vi "PicoScope6000aGetBlock.vi"(0 "handle in":i16, 1 "Acquisition Settings":T3 {"postTriggerSamples" format="%_6p"; "preTriggerSamples" format="%_6p"}, 2 "Buffer and Transfer Settings":T1 {"Down-Sample Mode" items=["None", "Aggregate", "Decimate", "Average"]; "Down Sample Ratio" step=1; "Samples" format="%_6p"}, 3 "enabled array":i16[](array[numeric]), 7 "stop IsReady":bool, 11 "error in (no error)":errorcluster) -> (4 "handle out":i16, 6 "Buffers (Max or non-aggregated)":T2, 10 "Min Buffers":T2, 12 "noOfSamples":u64, 14 "overflow":i16, 15 "error out":errorcluster)   [LabVIEW 2009]
doc: "GetBlock calls RunBlock and Sets up data buffers then calls GetValues"
uses:
  ps6000a.dll
panel:
  in  "PicoAction 2":u32(ring) items=["NONE", "CLEAR_ALL", "ADD", "CLEAR_THIS_DATA_BUFFER", "CLEAR_WAVEFORM_DATA_BUFFERS", "CLEAR_WAVEFORM_READ_DATA_BUFFERS"]
  in  "PicoAction 1":u32(ring) items=["NONE", "CLEAR_ALL", "ADD", "CLEAR_THIS_DATA_BUFFER", "CLEAR_WAVEFORM_DATA_BUFFERS", "CLEAR_WAVEFORM_READ_DATA_BUFFERS"]
  # "Pico Buffer Actions"
  # "Samples can be equal to or less\nTotal Pre and Post Trigger Samples"
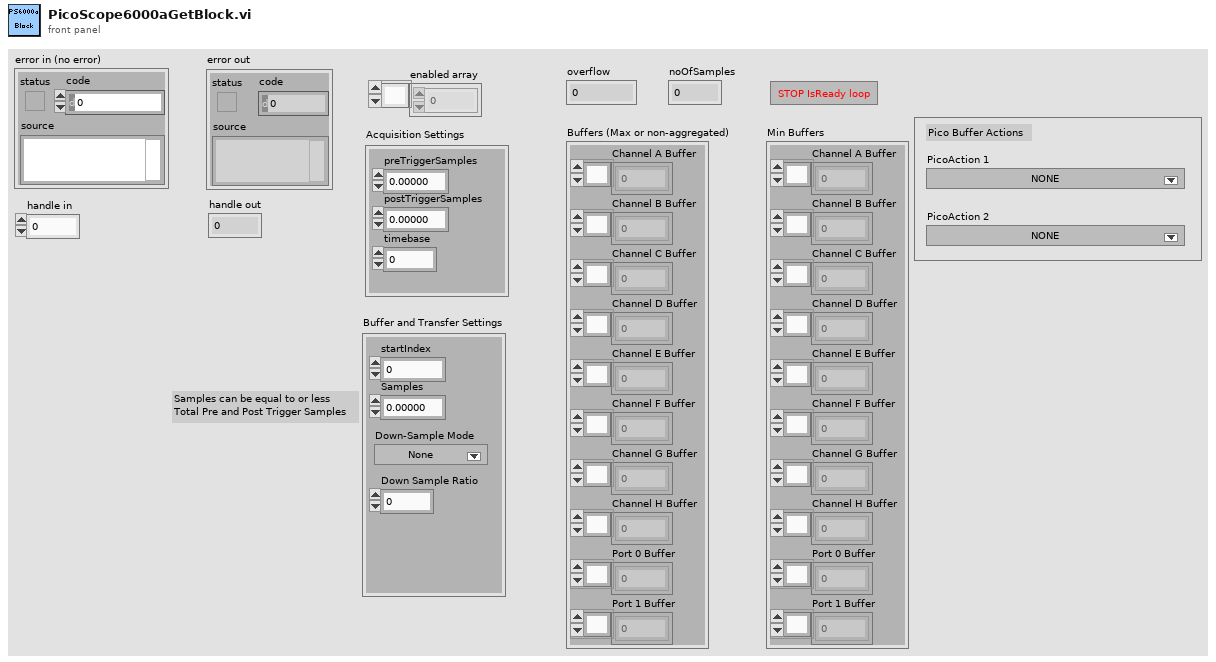
[diagram p1: front panel]
types:
  T1 = cluster{"startIndex":u64, "Samples":u64, "Down Sample Ratio":u64, "Down-Sample Mode":u32}
  T2 = cluster{"Channel A Buffer":i16[], "Channel B Buffer":i16[], "Channel C Buffer":i16[], "Channel D Buffer":i16[], "Channel E Buffer":i16[], "Channel F Buffer":i16[], "Channel G Buffer":i16[], "Channel H Buffer":i16[], "Port 0 Buffer":i16[], "Port 1 Buffer":i16[]}
  T3 = cluster{"preTriggerSamples":u64, "postTriggerSamples":u64, "timebase":u32}
  T4 = enum32{"PICO_INT8_T", "PICO_INT16_T", "PICO_INT32_T", "PICO_UINT32_T", "PICO_INT64_T", ""}
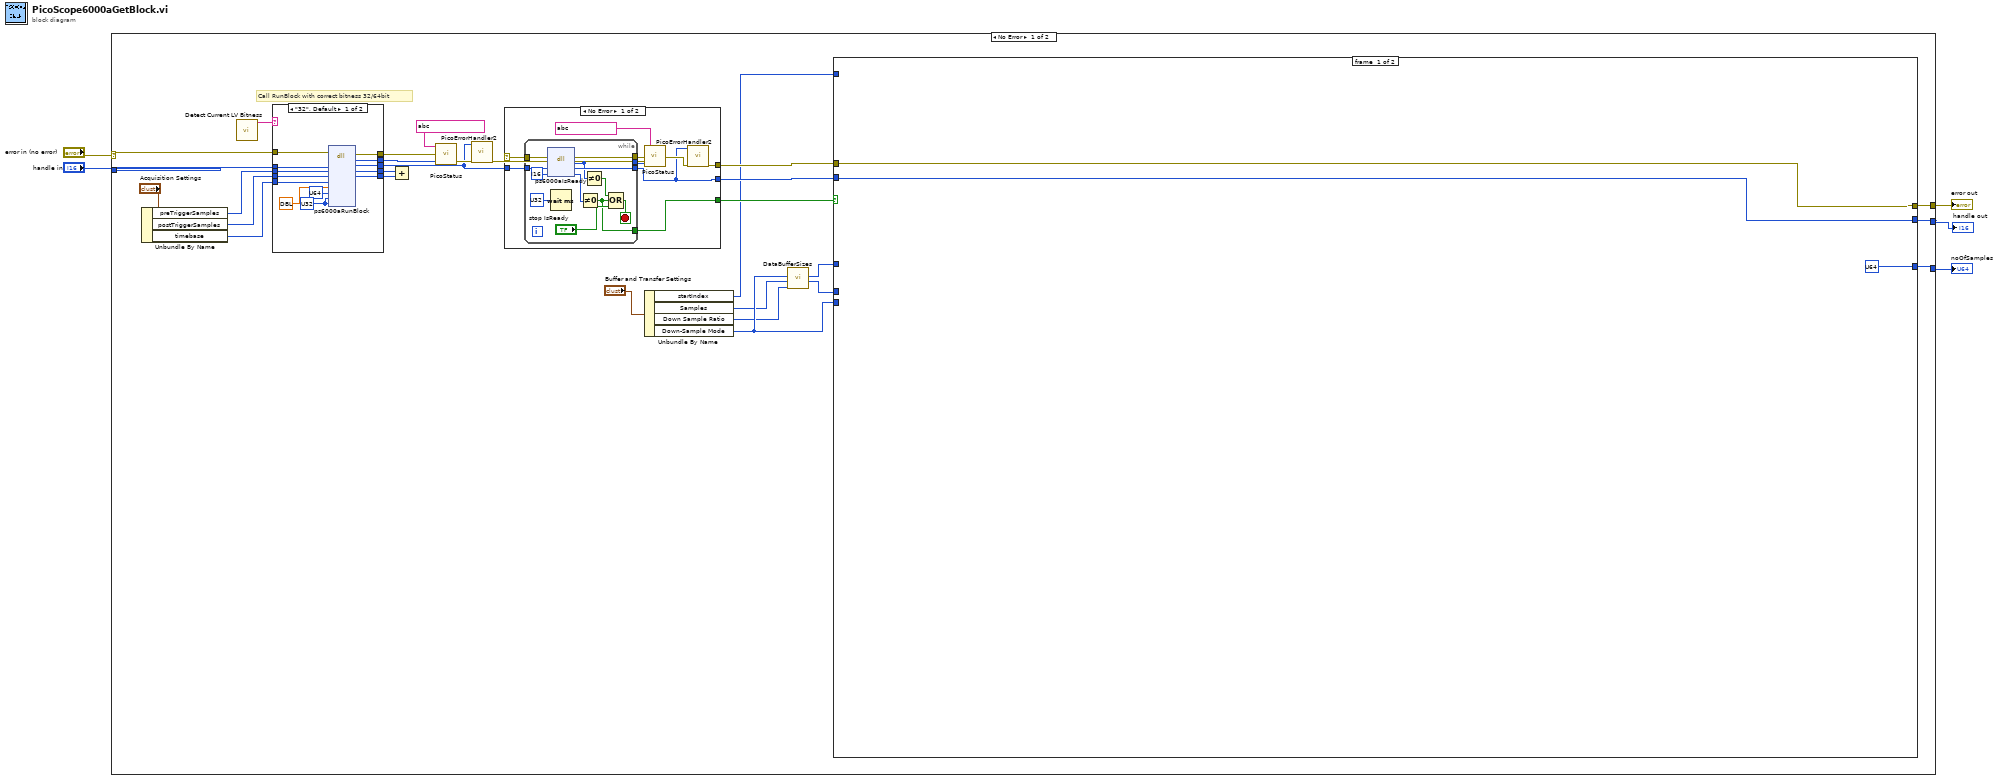
[diagram p0: block diagram]
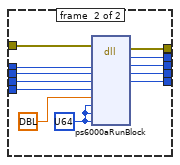
[diagram p2: hidden frame]
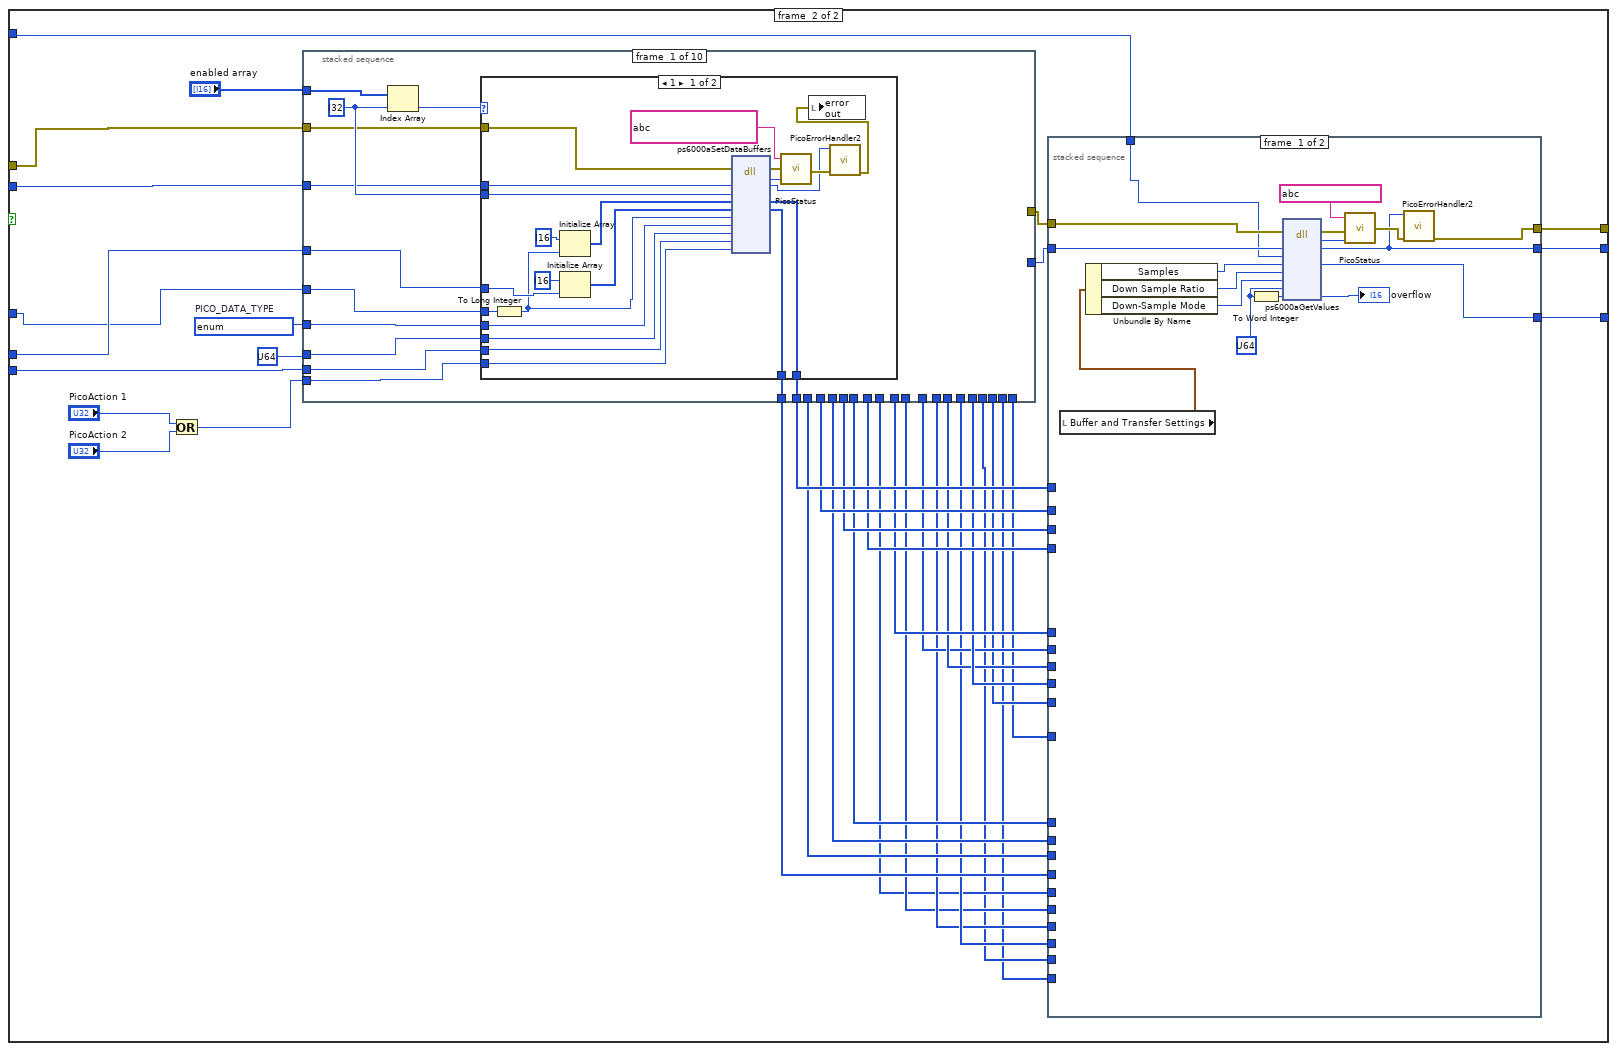
[diagram p3: hidden frame]
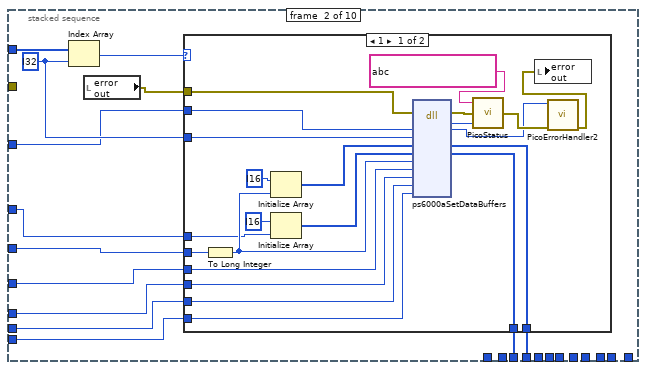
[diagram p5: hidden frame]
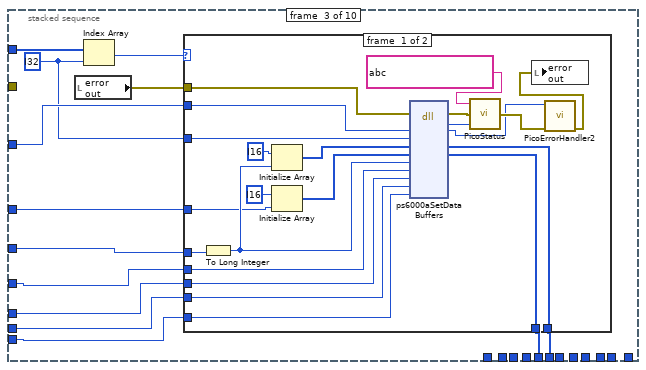
[diagram p7: hidden frame]
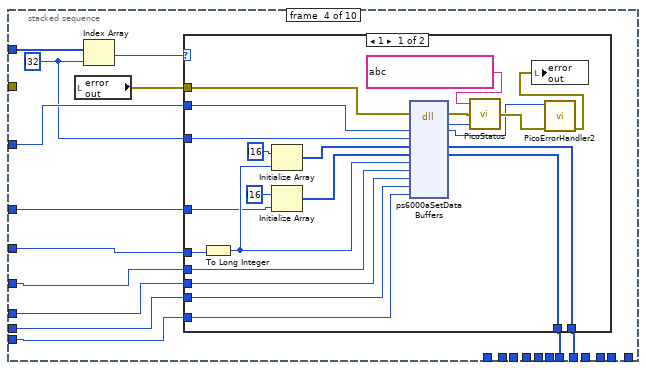
[diagram p9: hidden frame]
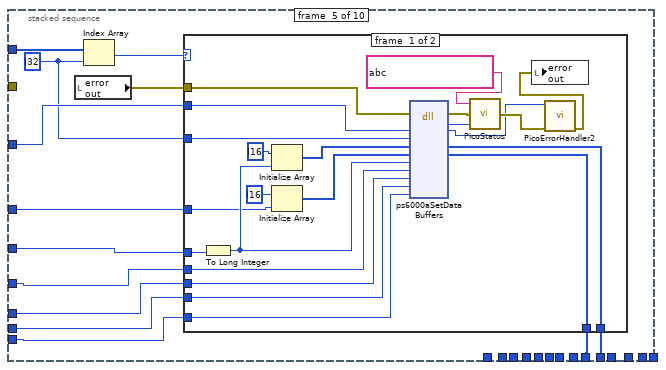
[diagram p11: hidden frame]
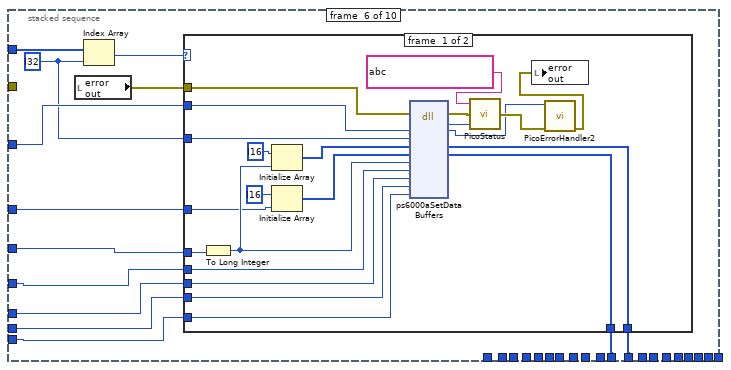
[diagram p13: hidden frame]
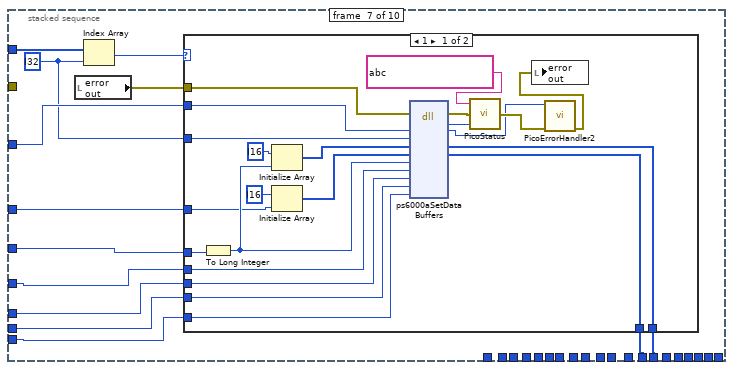
[diagram p15: hidden frame]
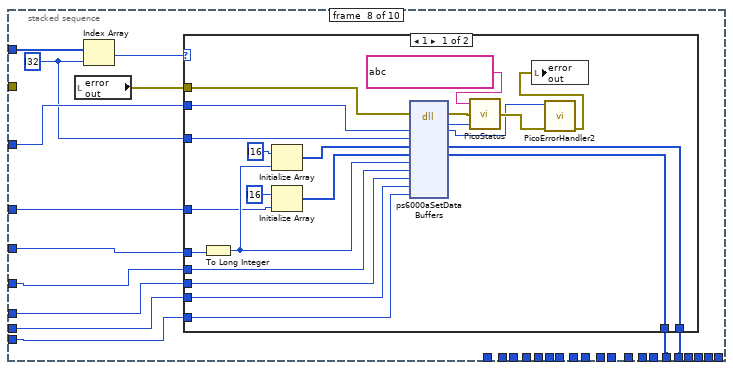
[diagram p17: hidden frame]
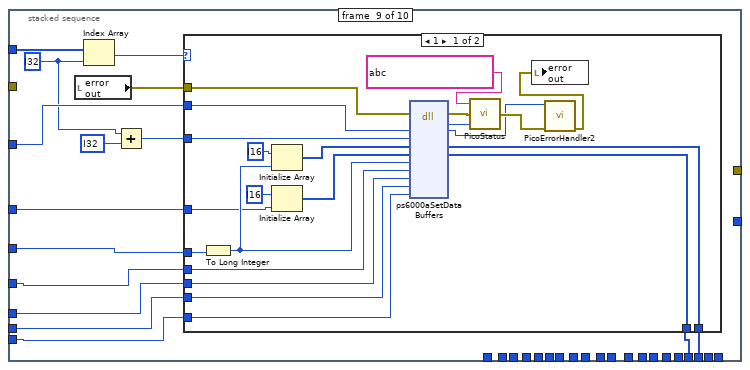
[diagram p19: hidden frame]
diagram:
  n1 = case shown="No Error" "error in (no error)" {
    selector: "error in (no error)" -> [w26 w524]
    tunnel: [w27 w524] -> w5
    tunnel: "handle in" -> [w25 w523]
    tunnel: [w24 w523] -> w4
    tunnel: [w19 u32 ? ("noOfSamples")] -> w1
    frame #0 {
      # "Call RunBlock with correct bitness 32/64bit"
      n2 = Unbundle By Name("Acquisition Settings") -> ("preTriggerSamples"=w23:u64, "postTriggerSamples"=w22:u64, "timebase"=w21:u32)
      n3 = call "Detect Current LV Bitness.vi"() -> ("bitness"=w11:string)  [unwired: 11 in]
      n4 = case shown="\"32\", Default" w11 {
        tunnel: [w46 w58] -> w33
        tunnel: [w45 w57] -> w32
        tunnel: [w44 w56] -> w30
        tunnel: [w43 w55] -> w29
        tunnel: w26 -> [w42 w54]
        tunnel: w25 -> [w41 w53]
        tunnel: w23 -> [w39 w51]
        tunnel: w22 -> [w38 w50]
        tunnel: w21 -> [w37 w49]
        tunnel: [w36 w48] -> w15
        frame #0 {
          w35 = u32 ? ("pParameter")
          n5 = dll-call lib="ps6000a.dll" fn="ps6000aRunBlock" ("ps3000.dll:_ps3000_open_unit@0")(error in=w42, "handle"=w41, "noOfPreTriggerSamples"=w39, "noOfPostTriggerSamples"=w38, "timebase"=w37, "timeIndisposedMs"=dbl ? ("pParameter"), "segmentIndex"=u64 ?, "lpReady"=w35, "pParameter"=w35) -> (error out=w43:errorcluster, "PICO_STATUS"=w44:u32, "handle"=w36:i16, "noOfPreTriggerSamples"=w46:u64, "noOfPostTriggerSamples"=w45:u64)  [unwired: 7 in, 1 out]
        }
        frame #1 {
          w47 = u64 ? ("pParameter")
          n6 = dll-call lib="ps6000a.dll" fn="ps6000aRunBlock" ("ps3000.dll:_ps3000_open_unit@0")(error in=w54, "handle"=w53, "noOfPreTriggerSamples"=w51, "noOfPostTriggerSamples"=w50, "timebase"=w49, "timeIndisposedMs"=dbl ? ("pParameter"), "segmentIndex"=w47, "lpReady"=w47, "pParameter"=w47) -> (error out=w55:errorcluster, "PICO_STATUS"=w56:u32, "handle"=w48:i16, "noOfPreTriggerSamples"=w58:u64, "noOfPostTriggerSamples"=w57:u64)  [unwired: 7 in, 1 out]
        }
      }
      n7 = Add(x=w33, y=w32) -> ()  [unwired: 1 out]
      n8 = call "PicoStatus.vi"("PICO STATUS"=w30, "error in"=w29, "source"=string ?) -> ("error out"=w20:errorcluster)
      n9 = call "PicoErrorHandler2.vi"("error in (no error)"=w20, "handle In"=w15) -> ("error out"=w18:errorcluster)  [unwired: 9 in]
      n10 = case shown="No Error" w18 {
        selector: w18 -> [w505 w520]
        tunnel: w15 -> [w506 w521]
        tunnel: [w499 w521] -> w16
        tunnel: [w500 w520] -> w17
        tunnel: [w498 bool ?] -> w14
        frame #0 {
          n11 = while {
            tunnel: [w518] -> w499
            tunnel: w506 -> [w517]
            tunnel: [w514] -> w503
            tunnel: w505 -> [w513]
            tunnel: [w512] -> w504
            tunnel: [w507] -> w498
            stop <- w516 stop-if-true
            n12 = dll-call lib="ps6000a.dll" fn="ps6000aIsReady" ("ps3000.dll:_ps3000_open_unit@0")(error in=w513, "handle"=w517, "ready"=i16 ?) -> (error out=w512:errorcluster, "PICO_STATUS"=w514:u32, "handle"=w518:i16, "ready"=w508:i16)  [unwired: 2 in, 1 out]
            n13 = Wait (ms)(milliseconds to wait=u32 ?) -> ()  [unwired: 1 out]
            n14 = Not Equal To 0?(x=w508) -> (x != 0?=w507:bool)
            n15 = Not Equal To 0?(x=w514) -> (x != 0?=w515:bool)
            n16 = Compound Arithmetic op=OR(w515, w507, "stop IsReady") -> (w516:bool)
          }
          n17 = call "PicoStatus.vi"("PICO STATUS"=w503, "error in"=w504, "source"=string ?) -> ("error out"=w501:errorcluster)
          n18 = call "PicoErrorHandler2.vi"("error in (no error)"=w501, "handle In"=w499) -> ("error out"=w500:errorcluster)  [unwired: 9 in]
        }
        frame #1 {
        }
      }
      n19 = Unbundle By Name("Buffer and Transfer Settings") -> ("startIndex"=w12:u64, "Samples"=w7:u64, "Down Sample Ratio"=w6:u64, "Down-Sample Mode"=w8:u32)
      n20 = call "DataBufferSizes.vi"("Down Sample Ratio"=w6, "Number of Samples"=w7, "Down-Sample Mode"=w8) -> ("min Buffer Size"=w9:i32, "Max Buffer Size"=w10:i32)  [unwired: 7 in]
      n21 = case shown="True" w14 {
        tunnel: [w59 w98] -> w27
        tunnel: [w60 w97] -> w24
        tunnel: [u64 ? ("noOfSamples") w96] -> w19
        tunnel: w17 -> [w59 w95]
        tunnel: w16 -> [w60 w94]
        tunnel: w9 -> [_ w67]
        tunnel: w10 -> [_ w62]
        tunnel: w8 -> [_ w93]
        tunnel: w12 -> [_ w68]
        frame #0 {
        }
        frame #1 {
          w69 = T4 ?  # PICO_DATA_TYPE
          n22 = Or(x="PicoAction 1", y="PicoAction 2") -> (x .or. y?=w70:u32)
          n23 = stacked-sequence {
            tunnel: "enabled array" -> [w110 w144 w180 w215 w250 w285 w320 w355 w392 w431]
            tunnel: w95 -> [w108 _ _ _ _ _ _ _ _ _]
            tunnel: w94 -> [w107 w143 w179 w214 w249 w284 w319 w354 w391 w430]
            tunnel: w62 -> [w106 w142 w170 w207 w242 w277 w312 w347 w385 w424]
            tunnel: w93 -> [w105 w136 w173 w210 w245 w280 w315 w350 w388 w427]
            tunnel: [w104 _ _ _ _ _ _ _ _ _] -> w91
            tunnel: [w103 _ _ _ _ _ _ _ _ _] -> w90
            tunnel: [_ w141 _ _ _ _ _ _ _ _] -> w89
            tunnel: [_ w140 _ _ _ _ _ _ _ _] -> w88
            tunnel: [_ _ w177 _ _ _ _ _ _ _] -> w87
            tunnel: [_ _ w176 _ _ _ _ _ _ _] -> w86
            tunnel: [_ _ _ w205 _ _ _ _ _ _] -> w85
            tunnel: [_ _ _ w204 _ _ _ _ _ _] -> w84
            tunnel: w69 -> [w102 w137 w171 w208 w243 w278 w313 w348 w386 w425]
            tunnel: u64 ? ("waveform") -> [w101 w135 w172 w209 w244 w279 w314 w349 w387 w426]
            tunnel: w70 -> [w100 w138 w174 w211 w246 w281 w316 w351 w389 w428]
            tunnel: [_ _ _ _ w239 _ _ _ _ _] -> w82
            tunnel: [_ _ _ _ _ _ _ w344 _ _] -> w81
            tunnel: [_ _ _ _ _ _ w309 _ _ _] -> w80
            tunnel: [_ _ _ _ _ w274 _ _ _ _] -> w79
            tunnel: [_ _ _ _ _ _ _ _ _ w422] -> w78
            tunnel: [_ _ _ _ _ _ _ _ _ w421] -> w77
            tunnel: [_ _ _ _ _ _ _ w345 _ _] -> w76
            tunnel: [_ _ _ _ _ _ w310 _ _ _] -> w75
            tunnel: [_ _ _ _ _ w275 _ _ _ _] -> w74
            tunnel: [_ _ _ _ w240 _ _ _ _ _] -> w73
            tunnel: w67 -> [w99 w134 w169 w206 w241 w276 w311 w346 w384 w423]
            tunnel: [_ _ _ _ _ _ _ _ w380 _] -> w66
            tunnel: [_ _ _ _ _ _ _ _ w379 _] -> w65
            tunnel: [_ _ _ _ _ _ _ _ _ w417] -> w64
            tunnel: [_ _ _ _ _ _ _ _ _ w416] -> w63
            frame #0 {
              w111 = i32 ? ("dimension size")
              n24 = Index Array(array=w110, index=w111) -> (element=w109:i16)
              n25 = case shown="1" w109 {
                tunnel: w111 -> [w128 _]
                tunnel: w108 -> [w133 _]
                tunnel: w107 -> [w130 _]
                tunnel: w106 -> [w113 _]
                tunnel: w105 -> [w122 _]
                tunnel: [w127 _] -> w104
                tunnel: [w126 _] -> w103
                tunnel: w102 -> [w121 _]
                tunnel: w101 -> [w120 _]
                tunnel: w100 -> [w119 _]
                tunnel: w99 -> [w115 _]
                frame #0 {
                  n26 = To Long Integer(number=w113) -> (32bit integer=w112:i32)
                  n27 = Initialize Array(i16 ? ("element"), w112) -> (w116:i16[])
                  n28 = Initialize Array(i16 ? ("element"), w115) -> (w114:i16[])
                  n29 = dll-call lib="ps6000a.dll" fn="ps6000aSetDataBuffers" ("ps3000.dll:_ps3000_open_unit@0")(error in=w133, "handle"=w130, "channel"=w128, "bufferMax"=w116, "bufferMin"=w114, "nSamples"=w112, "dataType"=w121, "waveform"=w120, "downSampleRatioMode"=w122, "action"=w119) -> (error out=w132:errorcluster, "PICO_STATUS"=w131:u32, "handle"=w123:i16, "bufferMax"=w126:i16[], "bufferMin"=w127:i16[])  [unwired: 8 in, 1 out]
                  n30 = call "PicoStatus.vi"("PICO STATUS"=w131, "error in"=w132, "source"=string ?) -> ("error out"=w125:errorcluster)
                  n31 = call "PicoErrorHandler2.vi"("error in (no error)"=w125, "handle In"=w123) -> ("error out"=w124:errorcluster)  [unwired: 9 in]
                  n32 = local write "error out"(w124) -> ()
                }
                frame #1 {
                }
              }
            }
            frame #1 {
              w146 = i32 ? ("dimension size")
              n33 = Index Array(array=w144, index=w146) -> (element=w145:i16)
              n34 = local read "error out"() -> (w139:errorcluster)
              n35 = case shown="1" w145 {
                tunnel: w146 -> [w148 _]
                tunnel: w139 -> [w162 _]
                tunnel: w143 -> [w147 _]
                tunnel: w135 -> [w157 _]
                tunnel: w142 -> [w152 _]
                tunnel: [w160 _] -> w141
                tunnel: [w161 _] -> w140
                tunnel: w138 -> [w159 _]
                tunnel: w137 -> [w156 _]
                tunnel: w136 -> [w158 _]
                tunnel: w134 -> [w151 _]
                frame #0 {
                  n36 = To Long Integer(number=w152) -> (32bit integer=w153:i32)
                  n37 = Initialize Array(i16 ? ("element"), w153) -> (w149:i16[])
                  n38 = Initialize Array(i16 ? ("element"), w151) -> (w150:i16[])
                  n39 = dll-call lib="ps6000a.dll" fn="ps6000aSetDataBuffers" ("ps3000.dll:_ps3000_open_unit@0")(error in=w162, "handle"=w147, "channel"=w148, "bufferMax"=w149, "bufferMin"=w150, "nSamples"=w153, "dataType"=w156, "waveform"=w157, "downSampleRatioMode"=w158, "action"=w159) -> (error out=w165:errorcluster, "PICO_STATUS"=w164:u32, "handle"=w163:i16, "bufferMax"=w161:i16[], "bufferMin"=w160:i16[])  [unwired: 8 in, 1 out]
                  n40 = call "PicoStatus.vi"("PICO STATUS"=w164, "error in"=w165, "source"=string ?) -> ("error out"=w167:errorcluster)
                  n41 = call "PicoErrorHandler2.vi"("error in (no error)"=w167, "handle In"=w163) -> ("error out"=w166:errorcluster)  [unwired: 9 in]
                  n42 = local write "error out"(w166) -> ()
                }
                frame #1 {
                }
              }
            }
            frame #2 {
              w175 = i32 ? ("dimension size")
              n43 = local read "error out"() -> (w178:errorcluster)
              n44 = Index Array(array=w180, index=w175) -> (element=w181:i16)
              n45 = case shown="0, Default" w181 {
                tunnel: w178 -> [w195 _]
                tunnel: w179 -> [w194 _]
                tunnel: [w196 _] -> w177
                tunnel: [w197 _] -> w176
                tunnel: w175 -> [w193 _]
                tunnel: w174 -> [w188 _]
                tunnel: w173 -> [w187 _]
                tunnel: w172 -> [w186 _]
                tunnel: w171 -> [w185 _]
                tunnel: w170 -> [w184 _]
                tunnel: w169 -> [w182 _]
                frame #0 {
                  n46 = To Long Integer(number=w184) -> (32bit integer=w183:i32)
                  n47 = Initialize Array(i16 ? ("element"), w183) -> (w190:i16[])
                  n48 = Initialize Array(i16 ? ("element"), w182) -> (w189:i16[])
                  n49 = dll-call lib="ps6000a.dll" fn="ps6000aSetDataBuffers" ("ps3000.dll:_ps3000_open_unit@0")(error in=w195, "handle"=w194, "channel"=w193, "bufferMax"=w190, "bufferMin"=w189, "nSamples"=w183, "dataType"=w185, "waveform"=w186, "downSampleRatioMode"=w187, "action"=w188) -> (error out=w200:errorcluster, "PICO_STATUS"=w199:u32, "handle"=w198:i16, "bufferMax"=w197:i16[], "bufferMin"=w196:i16[])  [unwired: 8 in, 1 out]
                  n50 = call "PicoStatus.vi"("PICO STATUS"=w199, "error in"=w200, "source"=string ?) -> ("error out"=w202:errorcluster)
                  n51 = call "PicoErrorHandler2.vi"("error in (no error)"=w202, "handle In"=w198) -> ("error out"=w201:errorcluster)  [unwired: 9 in]
                  n52 = local write "error out"(w201) -> ()
                }
                frame #1 {
                }
              }
            }
            frame #3 {
              w212 = i32 ? ("dimension size")
              n53 = local read "error out"() -> (w213:errorcluster)
              n54 = Index Array(array=w215, index=w212) -> (element=w216:i16)
              n55 = case shown="1" w216 {
                tunnel: w213 -> [w230 _]
                tunnel: w214 -> [w229 _]
                tunnel: [w231 _] -> w205
                tunnel: [w232 _] -> w204
                tunnel: w212 -> [w228 _]
                tunnel: w211 -> [w223 _]
                tunnel: w210 -> [w222 _]
                tunnel: w209 -> [w221 _]
                tunnel: w208 -> [w220 _]
                tunnel: w207 -> [w219 _]
                tunnel: w206 -> [w217 _]
                frame #0 {
                  n56 = To Long Integer(number=w219) -> (32bit integer=w218:i32)
                  n57 = Initialize Array(i16 ? ("element"), w218) -> (w225:i16[])
                  n58 = Initialize Array(i16 ? ("element"), w217) -> (w224:i16[])
                  n59 = dll-call lib="ps6000a.dll" fn="ps6000aSetDataBuffers" ("ps3000.dll:_ps3000_open_unit@0")(error in=w230, "handle"=w229, "channel"=w228, "bufferMax"=w225, "bufferMin"=w224, "nSamples"=w218, "dataType"=w220, "waveform"=w221, "downSampleRatioMode"=w222, "action"=w223) -> (error out=w235:errorcluster, "PICO_STATUS"=w234:u32, "handle"=w233:i16, "bufferMax"=w232:i16[], "bufferMin"=w231:i16[])  [unwired: 8 in, 1 out]
                  n60 = call "PicoStatus.vi"("PICO STATUS"=w234, "error in"=w235, "source"=string ?) -> ("error out"=w237:errorcluster)
                  n61 = call "PicoErrorHandler2.vi"("error in (no error)"=w237, "handle In"=w233) -> ("error out"=w236:errorcluster)  [unwired: 9 in]
                  n62 = local write "error out"(w236) -> ()
                }
                frame #1 {
                }
              }
            }
            frame #4 {
              w247 = i32 ? ("dimension size")
              n63 = local read "error out"() -> (w248:errorcluster)
              n64 = Index Array(array=w250, index=w247) -> (element=w251:i16)
              n65 = case shown="0, Default" w251 {
                tunnel: w248 -> [w265 _]
                tunnel: w249 -> [w264 _]
                tunnel: [w266 _] -> w240
                tunnel: [w267 _] -> w239
                tunnel: w247 -> [w263 _]
                tunnel: w246 -> [w258 _]
                tunnel: w245 -> [w257 _]
                tunnel: w244 -> [w256 _]
                tunnel: w243 -> [w255 _]
                tunnel: w242 -> [w254 _]
                tunnel: w241 -> [w252 _]
                frame #0 {
                  n66 = To Long Integer(number=w254) -> (32bit integer=w253:i32)
                  n67 = Initialize Array(i16 ? ("element"), w253) -> (w260:i16[])
                  n68 = Initialize Array(i16 ? ("element"), w252) -> (w259:i16[])
                  n69 = dll-call lib="ps6000a.dll" fn="ps6000aSetDataBuffers" ("ps3000.dll:_ps3000_open_unit@0")(error in=w265, "handle"=w264, "channel"=w263, "bufferMax"=w260, "bufferMin"=w259, "nSamples"=w253, "dataType"=w255, "waveform"=w256, "downSampleRatioMode"=w257, "action"=w258) -> (error out=w270:errorcluster, "PICO_STATUS"=w269:u32, "handle"=w268:i16, "bufferMax"=w267:i16[], "bufferMin"=w266:i16[])  [unwired: 8 in, 1 out]
                  n70 = call "PicoStatus.vi"("PICO STATUS"=w269, "error in"=w270, "source"=string ?) -> ("error out"=w272:errorcluster)
                  n71 = call "PicoErrorHandler2.vi"("error in (no error)"=w272, "handle In"=w268) -> ("error out"=w271:errorcluster)  [unwired: 9 in]
                  n72 = local write "error out"(w271) -> ()
                }
                frame #1 {
                }
              }
            }
            frame #5 {
              w282 = i32 ? ("dimension size")
              n73 = local read "error out"() -> (w283:errorcluster)
              n74 = Index Array(array=w285, index=w282) -> (element=w286:i16)
              n75 = case shown="0, Default" w286 {
                tunnel: w283 -> [w300 _]
                tunnel: w284 -> [w299 _]
                tunnel: [w301 _] -> w275
                tunnel: [w302 _] -> w274
                tunnel: w282 -> [w298 _]
                tunnel: w281 -> [w293 _]
                tunnel: w280 -> [w292 _]
                tunnel: w279 -> [w291 _]
                tunnel: w278 -> [w290 _]
                tunnel: w277 -> [w289 _]
                tunnel: w276 -> [w287 _]
                frame #0 {
                  n76 = To Long Integer(number=w289) -> (32bit integer=w288:i32)
                  n77 = Initialize Array(i16 ? ("element"), w288) -> (w295:i16[])
                  n78 = Initialize Array(i16 ? ("element"), w287) -> (w294:i16[])
                  n79 = dll-call lib="ps6000a.dll" fn="ps6000aSetDataBuffers" ("ps3000.dll:_ps3000_open_unit@0")(error in=w300, "handle"=w299, "channel"=w298, "bufferMax"=w295, "bufferMin"=w294, "nSamples"=w288, "dataType"=w290, "waveform"=w291, "downSampleRatioMode"=w292, "action"=w293) -> (error out=w305:errorcluster, "PICO_STATUS"=w304:u32, "handle"=w303:i16, "bufferMax"=w302:i16[], "bufferMin"=w301:i16[])  [unwired: 8 in, 1 out]
                  n80 = call "PicoStatus.vi"("PICO STATUS"=w304, "error in"=w305, "source"=string ?) -> ("error out"=w307:errorcluster)
                  n81 = call "PicoErrorHandler2.vi"("error in (no error)"=w307, "handle In"=w303) -> ("error out"=w306:errorcluster)  [unwired: 9 in]
                  n82 = local write "error out"(w306) -> ()
                }
                frame #1 {
                }
              }
            }
            frame #6 {
              w317 = i32 ? ("dimension size")
              n83 = local read "error out"() -> (w318:errorcluster)
              n84 = Index Array(array=w320, index=w317) -> (element=w321:i16)
              n85 = case shown="1" w321 {
                tunnel: w318 -> [w335 _]
                tunnel: w319 -> [w334 _]
                tunnel: [w336 _] -> w310
                tunnel: [w337 _] -> w309
                tunnel: w317 -> [w333 _]
                tunnel: w316 -> [w328 _]
                tunnel: w315 -> [w327 _]
                tunnel: w314 -> [w326 _]
                tunnel: w313 -> [w325 _]
                tunnel: w312 -> [w324 _]
                tunnel: w311 -> [w322 _]
                frame #0 {
                  n86 = To Long Integer(number=w324) -> (32bit integer=w323:i32)
                  n87 = Initialize Array(i16 ? ("element"), w323) -> (w330:i16[])
                  n88 = Initialize Array(i16 ? ("element"), w322) -> (w329:i16[])
                  n89 = dll-call lib="ps6000a.dll" fn="ps6000aSetDataBuffers" ("ps3000.dll:_ps3000_open_unit@0")(error in=w335, "handle"=w334, "channel"=w333, "bufferMax"=w330, "bufferMin"=w329, "nSamples"=w323, "dataType"=w325, "waveform"=w326, "downSampleRatioMode"=w327, "action"=w328) -> (error out=w340:errorcluster, "PICO_STATUS"=w339:u32, "handle"=w338:i16, "bufferMax"=w337:i16[], "bufferMin"=w336:i16[])  [unwired: 8 in, 1 out]
                  n90 = call "PicoStatus.vi"("PICO STATUS"=w339, "error in"=w340, "source"=string ?) -> ("error out"=w342:errorcluster)
                  n91 = call "PicoErrorHandler2.vi"("error in (no error)"=w342, "handle In"=w338) -> ("error out"=w341:errorcluster)  [unwired: 9 in]
                  n92 = local write "error out"(w341) -> ()
                }
                frame #1 {
                }
              }
            }
            frame #7 {
              w352 = i32 ? ("dimension size")
              n93 = local read "error out"() -> (w353:errorcluster)
              n94 = Index Array(array=w355, index=w352) -> (element=w356:i16)
              n95 = case shown="1" w356 {
                tunnel: w353 -> [w370 _]
                tunnel: w354 -> [w369 _]
                tunnel: [w371 _] -> w345
                tunnel: [w372 _] -> w344
                tunnel: w352 -> [w368 _]
                tunnel: w351 -> [w363 _]
                tunnel: w350 -> [w362 _]
                tunnel: w349 -> [w361 _]
                tunnel: w348 -> [w360 _]
                tunnel: w347 -> [w359 _]
                tunnel: w346 -> [w357 _]
                frame #0 {
                  n96 = To Long Integer(number=w359) -> (32bit integer=w358:i32)
                  n97 = Initialize Array(i16 ? ("element"), w358) -> (w365:i16[])
                  n98 = Initialize Array(i16 ? ("element"), w357) -> (w364:i16[])
                  n99 = dll-call lib="ps6000a.dll" fn="ps6000aSetDataBuffers" ("ps3000.dll:_ps3000_open_unit@0")(error in=w370, "handle"=w369, "channel"=w368, "bufferMax"=w365, "bufferMin"=w364, "nSamples"=w358, "dataType"=w360, "waveform"=w361, "downSampleRatioMode"=w362, "action"=w363) -> (error out=w375:errorcluster, "PICO_STATUS"=w374:u32, "handle"=w373:i16, "bufferMax"=w372:i16[], "bufferMin"=w371:i16[])  [unwired: 8 in, 1 out]
                  n100 = call "PicoStatus.vi"("PICO STATUS"=w374, "error in"=w375, "source"=string ?) -> ("error out"=w377:errorcluster)
                  n101 = call "PicoErrorHandler2.vi"("error in (no error)"=w377, "handle In"=w373) -> ("error out"=w376:errorcluster)  [unwired: 9 in]
                  n102 = local write "error out"(w376) -> ()
                }
                frame #1 {
                }
              }
            }
            frame #8 {
              w381 = i32 ? ("dimension size")
              n103 = local read "error out"() -> (w390:errorcluster)
              n104 = Index Array(array=w392, index=w381) -> (element=w393:i16)
              n105 = Add(x=w381, y=i32 ?) -> (x+y=w382:i32)
              n106 = case shown="1" w393 {
                tunnel: w390 -> [w407 _]
                tunnel: w391 -> [w406 _]
                tunnel: [w408 _] -> w380
                tunnel: [w409 _] -> w379
                tunnel: w382 -> [w405 _]
                tunnel: w389 -> [w400 _]
                tunnel: w388 -> [w399 _]
                tunnel: w387 -> [w398 _]
                tunnel: w386 -> [w397 _]
                tunnel: w385 -> [w396 _]
                tunnel: w384 -> [w394 _]
                frame #0 {
                  n107 = To Long Integer(number=w396) -> (32bit integer=w395:i32)
                  n108 = Initialize Array(i16 ? ("element"), w395) -> (w402:i16[])
                  n109 = Initialize Array(i16 ? ("element"), w394) -> (w401:i16[])
                  n110 = dll-call lib="ps6000a.dll" fn="ps6000aSetDataBuffers" ("ps3000.dll:_ps3000_open_unit@0")(error in=w407, "handle"=w406, "channel"=w405, "bufferMax"=w402, "bufferMin"=w401, "nSamples"=w395, "dataType"=w397, "waveform"=w398, "downSampleRatioMode"=w399, "action"=w400) -> (error out=w412:errorcluster, "PICO_STATUS"=w411:u32, "handle"=w410:i16, "bufferMax"=w409:i16[], "bufferMin"=w408:i16[])  [unwired: 8 in, 1 out]
                  n111 = call "PicoStatus.vi"("PICO STATUS"=w411, "error in"=w412, "source"=string ?) -> ("error out"=w414:errorcluster)
                  n112 = call "PicoErrorHandler2.vi"("error in (no error)"=w414, "handle In"=w410) -> ("error out"=w413:errorcluster)  [unwired: 9 in]
                  n113 = local write "error out"(w413) -> ()
                }
                frame #1 {
                }
              }
            }
            frame #9 {
              w419 = i32 ? ("dimension size")
              n114 = local read "error out"() -> (w429:errorcluster)
              n115 = Index Array(array=w431, index=w419) -> (element=w432:i16)
              n116 = Add(x=w419, y=i32 ?) -> (x+y=w420:i32)
              n117 = case shown="1" w432 {
                tunnel: w429 -> [w448 w456]
                tunnel: w430 -> [w447 w455]
                tunnel: [w449 _] -> w417
                tunnel: [w450 _] -> w416
                tunnel: w420 -> [w446 _]
                tunnel: w428 -> [w441 _]
                tunnel: w427 -> [w440 _]
                tunnel: w426 -> [w439 _]
                tunnel: w425 -> [w438 _]
                tunnel: w424 -> [w437 _]
                tunnel: w423 -> [w435 _]
                tunnel: [w434 w456] -> w422
                tunnel: [w433 w455] -> w421
                frame #0 {
                  n118 = To Long Integer(number=w437) -> (32bit integer=w436:i32)
                  n119 = Initialize Array(i16 ? ("element"), w436) -> (w443:i16[])
                  n120 = Initialize Array(i16 ? ("element"), w435) -> (w442:i16[])
                  n121 = dll-call lib="ps6000a.dll" fn="ps6000aSetDataBuffers" ("ps3000.dll:_ps3000_open_unit@0")(error in=w448, "handle"=w447, "channel"=w446, "bufferMax"=w443, "bufferMin"=w442, "nSamples"=w436, "dataType"=w438, "waveform"=w439, "downSampleRatioMode"=w440, "action"=w441) -> (error out=w452:errorcluster, "PICO_STATUS"=w451:u32, "handle"=w433:i16, "bufferMax"=w450:i16[], "bufferMin"=w449:i16[])  [unwired: 8 in, 1 out]
                  n122 = call "PicoStatus.vi"("PICO STATUS"=w451, "error in"=w452, "source"=string ?) -> ("error out"=w453:errorcluster)
                  n123 = call "PicoErrorHandler2.vi"("error in (no error)"=w453, "handle In"=w433) -> ("error out"=w434:errorcluster)  [unwired: 9 in]
                }
                frame #1 {
                }
              }
            }
          }
          n124 = stacked-sequence {
            tunnel: [w462 _] -> w98
            tunnel: [w460 _] -> w97
            tunnel: [w465 _] -> w96
            tunnel: w91 -> [_ w486]
            tunnel: w90 -> [_ w497]
            tunnel: w89 -> [_ w487]
            tunnel: w88 -> [_ w496]
            tunnel: w87 -> [_ w488]
            tunnel: w86 -> [_ w495]
            tunnel: w85 -> [_ w489]
            tunnel: w84 -> [_ w494]
            tunnel: w78 -> [w464 _]
            tunnel: w77 -> [w463 _]
            tunnel: w82 -> [_ w493]
            tunnel: w81 -> [_ w492]
            tunnel: w80 -> [_ w491]
            tunnel: w79 -> [_ w490]
            tunnel: w76 -> [_ w485]
            tunnel: w75 -> [_ w484]
            tunnel: w74 -> [_ w483]
            tunnel: w73 -> [_ w482]
            tunnel: w68 -> [w457 _]
            tunnel: w66 -> [_ w481]
            tunnel: w65 -> [_ w480]
            tunnel: w64 -> [_ w479]
            tunnel: w63 -> [_ w478]
            frame #0 {
              w472 = u64 ? ("overflow")
              n125 = local read "Buffer and Transfer Settings"() -> (w459:T1)
              n126 = Unbundle By Name(w459) -> ("Samples"=w458:u64, "Down Sample Ratio"=w468:u64, "Down-Sample Mode"=w467:u32)
              n127 = To Word Integer(number=w472) -> (16bit integer=w466:i16)
              n128 = dll-call lib="ps6000a.dll" fn="ps6000aGetValues" ("ps3000.dll:_ps3000_open_unit@0")(error in=w464, "handle"=w463, "startIndex"=w457, "noOfSamples"=w458, "downSampleRatio"=w468, "downSampleRatioMode"=w467, "segmentIndex"=w472, "overflow"=w466) -> (error out=w470:errorcluster, "PICO_STATUS"=w471:u32, "handle"=w460:i16, "noOfSamples"=w465:u64, "overflow"=→"overflow":i16)  [unwired: 6 in, 1 out]
              n129 = call "PicoStatus.vi"("PICO STATUS"=w471, "error in"=w470, "source"=string ?) -> ("error out"=w461:errorcluster)
              n130 = call "PicoErrorHandler2.vi"("error in (no error)"=w461, "handle In"=w460) -> ("error out"=w462:errorcluster)  [unwired: 9 in]
            }
            frame #1 {
              n131 = Bundle By Name(cluster=T2 ? ("Min Buffers"), "Channel A Buffer"=w489, "Channel B Buffer"=w488, "Channel C Buffer"=w487, "Channel D Buffer"=w486, "Channel E Buffer"=w482, "Channel F Buffer"=w483, "Channel G Buffer"=w484, "Channel H Buffer"=w485, "Port 0 Buffer"=w481, "Port 1 Buffer"=w479) -> (→"Min Buffers":T2)
              n132 = Bundle By Name(cluster=T2 ? ("Buffers (Max or non-aggregated)"), "Channel A Buffer"=w497, "Channel B Buffer"=w496, "Channel C Buffer"=w495, "Channel D Buffer"=w494, "Channel E Buffer"=w493, "Channel F Buffer"=w490, "Channel G Buffer"=w491, "Channel H Buffer"=w492, "Port 0 Buffer"=w480, "Port 1 Buffer"=w478) -> (→"Buffers (Max or non-aggregated)":T2)
            }
          }
        }
      }
    }
    frame #1 {
    }
  }
  "error out" <- w5
  "handle out" <- w4
  "noOfSamples" <- w1
